vi "Zielscheibe.vi"() -> ()   [LabVIEW 2010]
panel:
  out "XY Graph":cluster{dbl[], dbl[]}[](graph)
  in  "Anzahl Schüsse":dbl
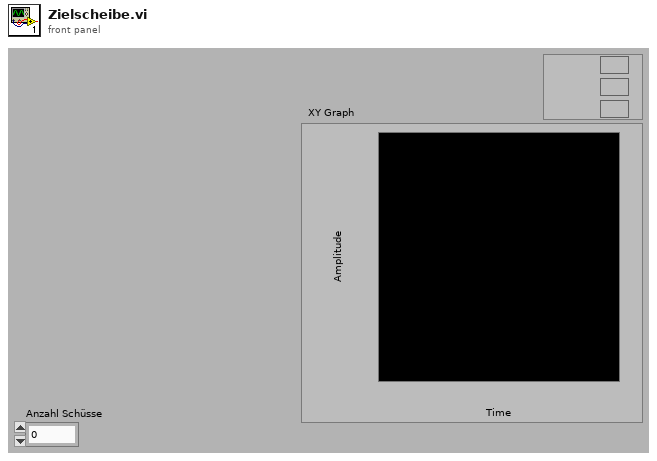
[diagram p1: front panel]
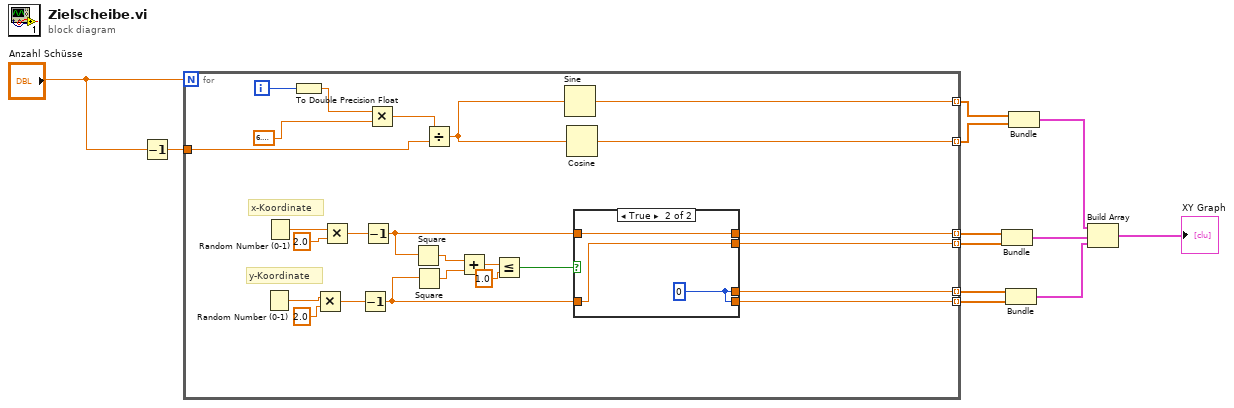
[diagram p0: block diagram]
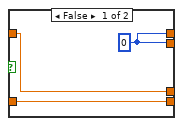
[diagram p2: hidden frame]
diagram:
  n1 = Decrement(x="Anzahl Schüsse") -> (x-1=w12:dbl)
  n2 = for {
    N: "Anzahl Schüsse" -> [_]
    tunnel: w12 -> [w19]
    tunnel: [w21] -> w10 mode=indexing
    tunnel: [w20] -> w9 mode=indexing
    tunnel: [w16] -> w6 mode=indexing
    tunnel: [w15] -> w4 mode=indexing
    tunnel: [w14] -> w3 mode=indexing
    tunnel: [w13] -> w5 mode=indexing
    i -> [w37]
    # "y-Koordinate"
    # "x-Koordinate"
    n3 = Random Number (0-1)() -> (number: 0 to 1=w29:dbl)
    n4 = Random Number (0-1)() -> (number: 0 to 1=w31:dbl)
    n5 = To Double Precision Float(number=w37) -> (double precision float=w36:dbl)
    n6 = Multiply(x=w29, y=2.0) -> (x*y=w27:dbl)
    n7 = Multiply(x=w31, y=2.0) -> (x*y=w28:dbl)
    n8 = Decrement(x=w27) -> (x-1=w18:dbl)
    n9 = Decrement(x=w28) -> (x-1=w17:dbl)
    n10 = Multiply(x=w36, y=6.283185307179586) -> (x*y=w34:dbl)
    n11 = Square(x=w17) -> (x^2=w26:dbl)
    n12 = Square(x=w18) -> (x^2=w25:dbl)
    n13 = Divide(x=w34, y=w19) -> (x/y=w33:dbl)
    n14 = Add(x=w26, y=w25) -> (x+y=w24:dbl)
    n15 = Less Or Equal?(x=w24, y=1.0) -> (x <= y?=w22:bool)
    n16 = Sine(x=w33) -> (sin(x)=w21:dbl)
    n17 = Cosine(x=w33) -> (cos(x)=w20:dbl)
    n18 = case shown="True" w22 {
      tunnel: w18 -> [w39 w42]
      tunnel: w17 -> [w40 w43]
      tunnel: [w38 w43] -> w16
      tunnel: [w40 w41] -> w15
      tunnel: [w39 w41] -> w14
      tunnel: [w38 w42] -> w13
      frame False {
        w38 = 0
      }
      frame True {
        w41 = 0
      }
    }
  }
  n19 = Bundle(w6, w5) -> (w2:cluster{dbl[], dbl[]})  [unwired: 1 in]
  n20 = Bundle(w4, w3) -> (w1:cluster{dbl[], dbl[]})  [unwired: 1 in]
  n21 = Bundle(w10, w9) -> (w8:cluster{dbl[], dbl[]})  [unwired: 1 in]
  n22 = Build Array(w8, w2, w1) -> (→"XY Graph":cluster{dbl[], dbl[]}[])
